vi "Arm Controller.vi"(8 "error in":errorcluster) -> ()   [LabVIEW 2019]
doc: "This VI executes continuously carrying out the current operation and responding to updates or new operations. It will often contain the timing or control code that is difficult to place directly in TeleOp. This VI generally opens all sensors and motors and isolates the rest of the robot code from knowing how the operations are carried out."
uses:
  <vilib>/Rock Robotics/WPI/Framework/Completion Status.ctl
  Arm Setpoints.ctl
  Arm Operations.ctl
  <vilib>/Rock Robotics/SystemInterfaces/DIO/FPGA_DIOChannel.ctl
  <vilib>/Rock Robotics/WPI/Encoder/WPI_EncoderType.ctl
  <vilib>/Rock Robotics/WPI/ThirdParty/Phoenix-LabVIEW/Motor Controller/Controls/CTRE_Phoenix_MotorControl_ControlMode.ctl
  <vilib>/Rock Robotics/WPI/Counter/WPI_CounterDigitalInputToDigitalSource.vi
  <vilib>/Rock Robotics/Network Tables/NT Write Boolean.vi
panel:
  in  "Interactive Values":T1
  out "Current\nCmd":string
  in  "Buttons":cluster{"Execute Cmd":bool, "Abort Cmd":bool}
  out "Command Timing":cluster{"Start Time (ms)":u32, "Iterations":i32}
  out "Status":T3
  # "Tip: It may be helpful to observe inputs and sensor values.\nYou may also want to display tuning or debugging controls."
  # "Interactive Command: You may fill in the settings for a command\nand schedule it with the Execute button. You can observe and abort\nany command while fine tuning the code for the controller."
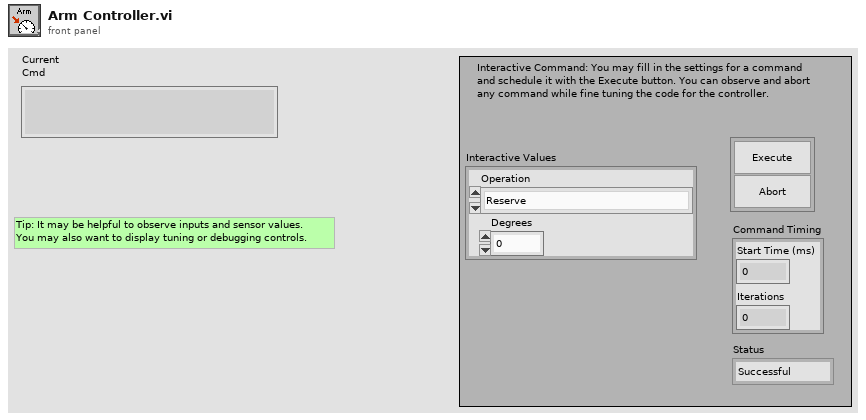
[diagram p1: front panel]
types:
  T1 = typedef "Arm Setpoints.ctl" = cluster{"Operation":T2, "Degrees":dbl}
  T2 = typedef "Arm Operations.ctl" = enum16{"Reserve", "Read Current", "bore_test", "Up", "Down", "Stop", "Up Reset", "Down Reset", "Immediate", ""}
  T3 = typedef "Completion Status.ctl" = enum16{"Successful", "Aborted", "Incomplete"}
  T4 = typedef "WPI_EncoderType.ctl" = enum16{"1x", "2x", "4x"}
  T5 = typedef "FPGA_DIOChannel.ctl" = enum8{"DIO 0", "DIO 1", "DIO 2", "DIO 3", "DIO 4", "DIO 5", "DIO 6", "DIO 7", "DIO 8", "DIO 9", "DIO MXP 0", "DIO MXP 1", "DIO MXP 2", "DIO MXP 3", "DIO MXP 4", "DIO MXP 5", "DIO MXP 6", "DIO MXP 7", "DIO MXP 8", "DIO MXP 9", "DIO MXP 10", "DIO MXP 11", "DIO MXP 12", "DIO MXP 13", "DIO MXP 14", "DIO MXP 15", "SPI Port CS1", "SPI Port CS2", "SPI Port CS3", "SPI Port MISO", "SPI Port MOSI", "Invalid"}
  T6 = typedef "WPI_MotorControlDeviceRef.ctl" = cluster{"DeviceStatus":errorcluster, "Type":T7, "PWM":cluster{"PWM Channel":T8, "DeadBand":T9}, "CAN":cluster{"Device Number":u8, "SetOutput VI Ref":variant, "GetOutput VI Ref":variant, "Enable VI Ref":variant, "Disable VI Ref":variant, "Data":variant}, "Invert":bool, "DIO PWM":cluster{"PWM \"Enable\" Channel":T8, "DIOChannel":T5, "PWM Rate":dbl}}
  T7 = typedef "WPI_MotorControlType.ctl" = enum16{"PWM", "CAN", "DIO PWM"}
  T8 = typedef "FPGA_DIOPWMChannel.ctl" = enum8{"PWM 0", "PWM 1", "PWM 2", "PWM 3", "PWM 4", "PWM 5", "PWM 6", "PWM 7", "PWM 8", "PWM 9", "PWM MXP 0", "PWM MXP 1", "PWM MXP 2", "PWM MXP 3", "PWM MXP 4", "PWM MXP 5", "PWM MXP 6", "PWM MXP 7", "PWM MXP 8", "PWM MXP 9", "Invalid"}
  T9 = typedef "WPI_PWMDeadband.ctl" = cluster{"Name":string, "maxPositivePwm":i32, "minPositivePwm":i32, "centerPwm":i32, "maxNegativePwm":i32, "minNegativePwm":i32, "angularRange":u16}
  T10 = typedef "WPI_DigitalInputDevRef.ctl" = cluster{"DevStatus":errorcluster, "DIO Channel":T5}
  T11 = typedef "FPGA_CounterEncoderSourceConvertionLVSourceType.ctl" = cluster{"DevStatus":errorcluster, "AnalogTriggerMode?":bool, "DigitalMode":cluster{"DIO Channel":T12}, "AnalogTriggerMode":cluster{"AnalogTriggerIndex":T13, "OutputType":T14}}
  T12 = typedef "FPGA_DIODigitalSourceChannel.ctl" = enum8{"DIO 0", "DIO 1", "DIO 2", "DIO 3", "DIO 4", "DIO 5", "DIO 6", "DIO 7", "DIO 8", "DIO 9", "DIO MXP 0", "DIO MXP 1", "DIO MXP 2", "DIO MXP 3", "DIO MXP 4", "DIO MXP 5", "DIO MXP 6", "DIO MXP 7", "DIO MXP 8", "DIO MXP 9", "DIO MXP 10", "DIO MXP 11", "DIO MXP 12", "DIO MXP 13", "DIO MXP 14", "DIO MXP 15", "SPI Port CS1", "SPI Port CS2", "SPI Port CS3", "SPI Port MISO", "SPI Port MOSI", "Disabled"}
  T13 = typedef "FPGA_AnalogTriggerIndex.ctl" = enum8{"Trig 0", "Trig 1", "Trig 2", "Trig 3", "Trig 4", "Trig 5", "Trig 6", "Trig 7", "Invalid"}
  T14 = typedef "FPGA_AnalogTriggerOutType.ctl" = enum16{"InWindow", "TriggerState", "Rising", "Falling"}
  T15 = typedef "WPI_EncoderDevRef.ctl" = cluster{"DevStatus":errorcluster, "EncoderIndex":T16, "CounterIndex":T17, "DistancePerCount":dbl, "Decoding Type":T4}
  T16 = typedef "FPGA_EncoderIdx.ctl" = enum8{"Enc 0", "Enc 1", "Enc 2", "Enc 3", "Enc 4", "Enc 5", "Enc 6", "Enc 7", "Invalid"}
  T17 = typedef "FPGA_CounterCtrSystemIndex.ctl" = enum8{"Ctr 0", "Ctr 1", "Ctr 2", "Ctr 3", "Ctr 4", "Ctr 5", "Ctr 6", "Ctr 7", "Invalid"}
  T18 = typedef "Command Status Info.ctl" = cluster{"Name":string, "Status":T3, "notifier out":T19}
  T19 = typedef "Completion Notifier.ctl" = refnum<notifier>
  T20 = cluster{"Current Command":T1, "Command Timing":cluster{"Start Time (ms)":u32, "Iterations":i32}, "Command Arguments":cluster{"Command Info":T18, "Description":string, "Default Command":T1, "queue out":refnum<queue>, "Subsystem Name":string}}
  T21 = typedef "CTRE_Phoenix_MotorControl_ControlMode.ctl" = u16
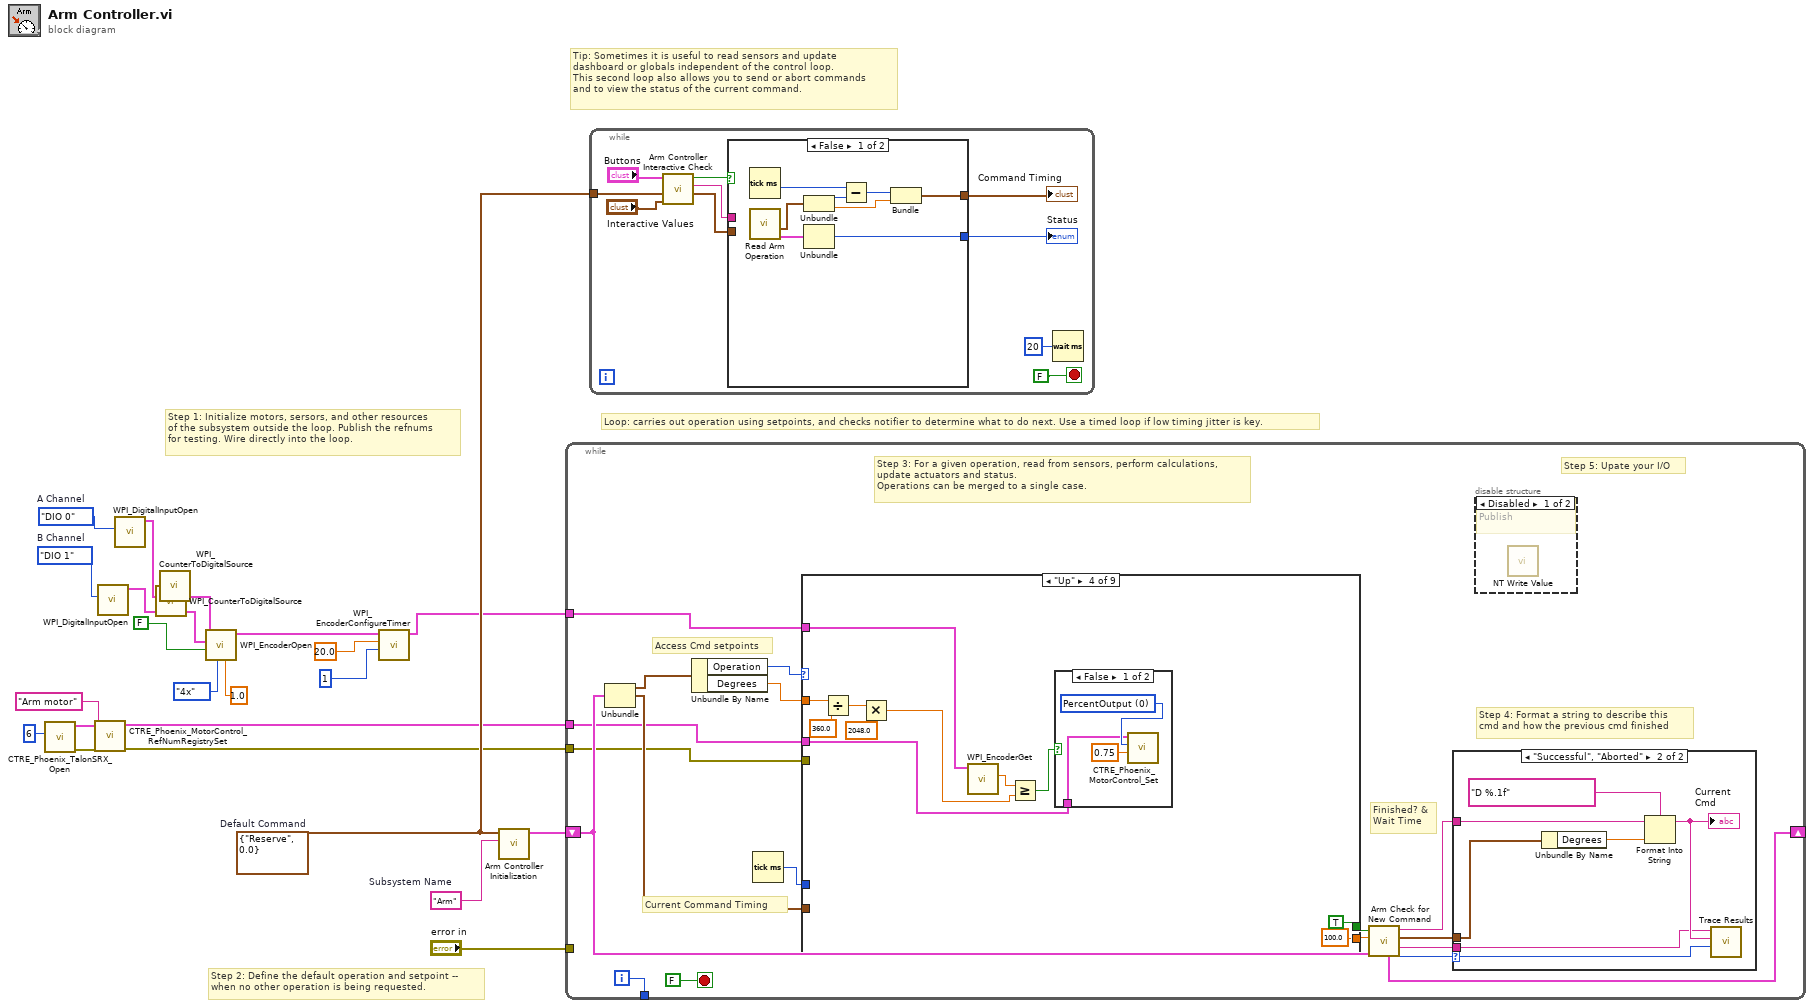
[diagram p0: block diagram]
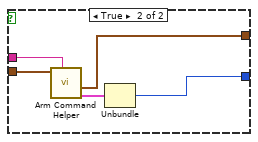
[diagram p2: hidden frame]
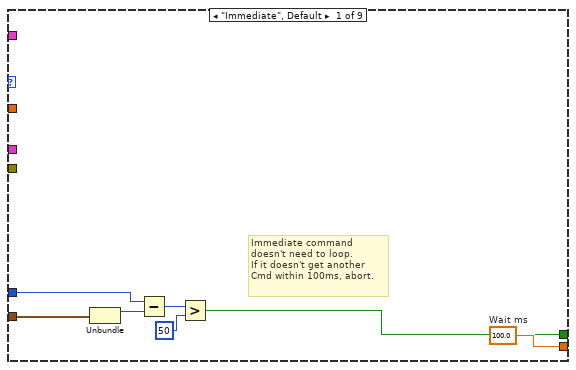
[diagram p5: hidden frame]
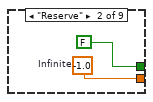
[diagram p6: hidden frame]
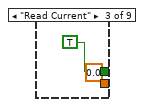
[diagram p7: hidden frame]
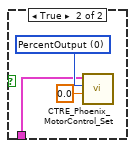
[diagram p8: hidden frame]
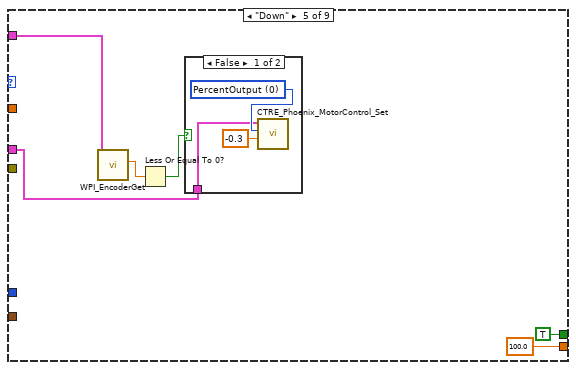
[diagram p9: hidden frame]
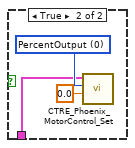
[diagram p10: hidden frame]
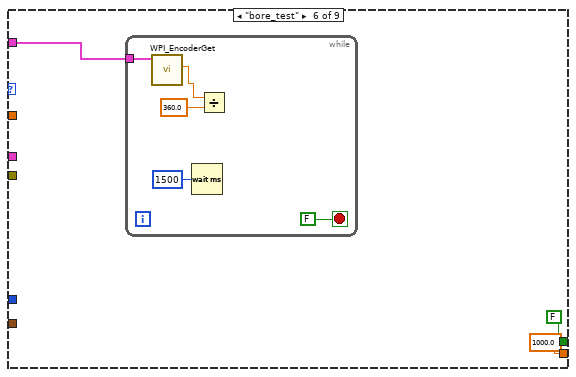
[diagram p11: hidden frame]
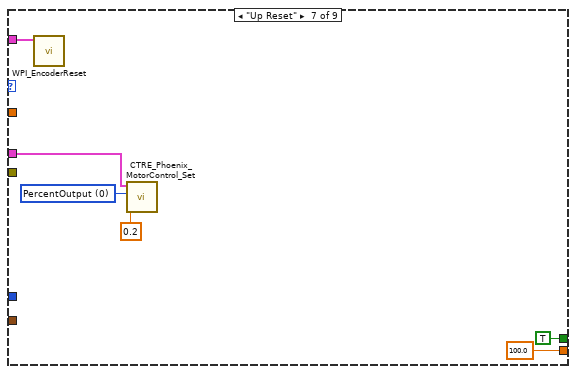
[diagram p12: hidden frame]
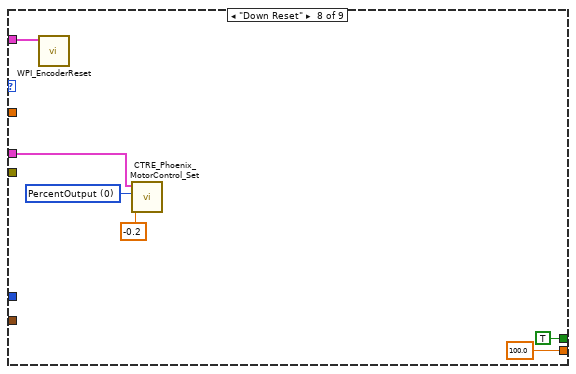
[diagram p13: hidden frame]
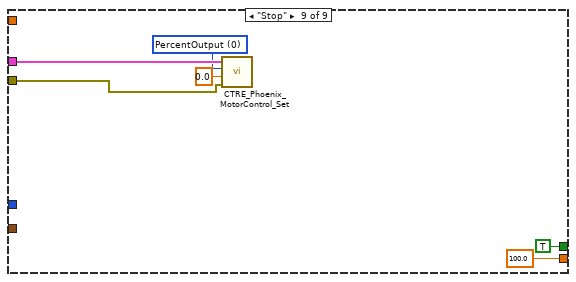
[diagram p14: hidden frame]
diagram:
  w19 = FPGA_DIOChannel."DIO 1"  # B Channel
  w18 = FPGA_DIOChannel."DIO 0"  # A Channel
  w20 = T1 {"Operation"=enum."Reserve", "Degrees"=0.0}  # Default Command
  w21 = "Arm"  # Subsystem Name
  # "Tip: Sometimes it is useful to read sensors and update\ndashboard or globals independent of the control loop.\nThis second loop also allows you to send or abort commands\nand to view the status of the current command."
  # "Step 2: Define the default operation and setpoint --\nwhen no other operation is being requested."
  # "Step 1: Initialize motors, sersors, and other resources\nof the subsystem outside the loop. Publish the refnums\nfor testing. Wire directly into the loop."
  # "Loop: carries out operation using setpoints, and checks notifier to determine what to do next. Use a timed loop if low timing jitter is key."
  n1 = call <vilib>:"CTRE_Phoenix_TalonSRX_Open.vi"("Device Number"=u8 6) -> ("error out"=w6:errorcluster, "CAN Talon SRX Ref"=w5:T6)  [unwired: 9 in]
  n2 = call <vilib>:"CTRE_Phoenix_MotorControl_RefNumRegistrySet.vi"("error in (no error)"=w6, "refnum name"="Arm motor", "PhoenixMotorControlDevRef"=w5) -> ("error out"=w2:errorcluster, "PhoenixMotorControlDevRef"=w3:T6)  [unwired: 7 in]
  n3 = call <vilib>:"WPI_DigitalInputOpen.vi"("DIO Channel"=w19) -> ("DigitalInputDevRef"=w16:T10)  [unwired: 1 in, 9 out]
  n4 = call <vilib>:"WPI_DigitalInputOpen.vi"("DIO Channel"=w18) -> ("DigitalInputDevRef"=w15:T10)  [unwired: 1 in, 9 out]
  n5 = call-poly <vilib>:"WPI_CounterToDigitalSource.vi"("DigitalInputDevRef"=w16) -> ("Digital Source"=w17:T11)  [unwired: 6 out]
  n6 = call-poly <vilib>:"WPI_CounterToDigitalSource.vi"("DigitalInputDevRef"=w15) -> ("Digital Source"=w14:T11)  [unwired: 6 out]
  n7 = call <vilib>:"WPI_EncoderOpen.vi"("DistancePerCount"=1.0, "Decoding Type"=WPI_EncoderType."4x", "Invert Direction (False)"=FALSE, "BSource"=w17, "ASource"=w14) -> ("EncoderDevRef"=w13:T15)  [unwired: 3 in, 3 out]
  n8 = call <vilib>:"WPI_EncoderConfigureTimer.vi"("Number Samples to Average"=u8 1, "Minimum Rate"=20.0, "EncoderDevRef"=w13) -> ("EncoderDevRef"=w12:T15)  [unwired: 7 in, 1 out]
  n9 = call "Arm Controller Initialization.vi"("Subsystem Name"=w21, "Default Command"=w20) -> ("Current Command"=w22:T20)  [unwired: 9 in]
  n10 = while {
    shift-right: [w36] -> _
    shift-left: w22 -> [w29]
    tunnel: [w40] -> _
    tunnel: "error in" -> [_]
    tunnel: w12 -> [w27]
    tunnel: w3 -> [w25]
    tunnel: w2 -> [w24]
    i -> [w40]
    stop <- FALSE stop-if-true
    # "Step 5: Upate your I/O"
    # "Step 4: Format a string to describe this\ncmd and how the previous cmd finished"
    # "Current Command Timing"
    # "Access Cmd setpoints"
    # "Finished? &\nWait Time"
    # "Step 3: For a given operation, read from sensors, perform calculations,\nupdate actuators and status.\nOperations can be merged to a single case."
    n11 = Unbundle(w29) -> ("Current Command"=w39:T1, "Command Timing"=w37:cluster{"Start Time (ms)":u32, "Iterations":i32})  [unwired: 1 out]
    n12 = Unbundle By Name(w39) -> ("Operation"=w26:T2, "Degrees"=w28:dbl)
    n13 = Tick Count (ms)() -> (millisecond timer value=w38:u32)
    n14 = case shown="\"Up\"" w26 {
      tunnel: [w55 w57 0.0 ("Infinite") 100.0 ("Infinite") 100.0 ("Infinite") 1000.0 ("Infinite") 100.0 ("Infinite") 100.0 ("Infinite") 100.0 ("Infinite")] -> w34
      tunnel: [w49 FALSE ("ignore previous (F)") TRUE TRUE ("ignore previous (F)") TRUE ("ignore previous (F)") FALSE ("ignore previous (F)") TRUE ("ignore previous (F)") TRUE ("ignore previous (F)") TRUE ("ignore previous (F)")] -> w35
      tunnel: w37 -> [w51 _ _ _ _ _ _ _ _]
      tunnel: w38 -> [w50 _ _ _ _ _ _ _ _]
      tunnel: w28 -> [_ _ _ w65 _ _ _ _ _]
      tunnel: w27 -> [_ _ _ w67 w80 w91 w99 w105 _]
      tunnel: w25 -> [_ _ _ w66 w79 _ w101 w106 w114]
      tunnel: w24 -> [_ _ _ _ _ _ _ _ w111]
      frame "Immediate", Default {
        w55 = 100.0  # Wait ms
        # "Immediate command\ndoesn't need to loop.\nIf it doesn't get another\nCmd within 100ms, abort."
        n15 = Unbundle(w51) -> ("Start Time (ms)"=w54:u32)  [unwired: 1 out]
        n16 = Subtract(x=w50, y=w54) -> (x-y=w53:u32)
        n17 = Greater?(x=w53, y=u8 50 ("Left Motor")) -> (0:w49:bool)
      }
      frame "Reserve" {
        w57 = -1.0  # Infinite
      }
      frame "Read Current" {
      }
      frame "Up" {
        n18 = Divide(x=w65, y=360.0) -> (x/y=w63:dbl)
        n19 = Multiply(x=w63, y=2048.0) -> (x*y=w61:dbl)
        n20 = call <vilib>:"WPI_EncoderGet.vi"("EncoderDevRef"=w67) -> ("Distance"=w69:dbl)  [unwired: 5 in, 5 out]
        n21 = Greater Or Equal?(x=w69, y=w61) -> (x >= y?=w68:bool)
        n22 = case shown="False" w68 {
          tunnel: w66 -> [w71 w74]
          frame False {
            w72 = T21 0 items=["PercentOutput"=0, "Position"=1, "Velocity"=2, "Current"=3, "Follower"=5, "MotionProfile"=6, "MotionMagic"=7, "MotionProfileArc"=10, "Disabled"=15] ("Control Mode")
            n23 = call <vilib>:"CTRE_Phoenix_MotorControl_Set.vi"("Output"=0.75, "Control Mode"=w72, "PhoenixMotorControlDevRef"=w71) -> ()  [unwired: 7 in, 2 out]
          }
          frame True {
            w76 = T21 0 items=["PercentOutput"=0, "Position"=1, "Velocity"=2, "Current"=3, "Follower"=5, "MotionProfile"=6, "MotionMagic"=7, "MotionProfileArc"=10, "Disabled"=15] ("Control Mode")
            n24 = call <vilib>:"CTRE_Phoenix_MotorControl_Set.vi"("Output"=0.0, "Control Mode"=w76, "PhoenixMotorControlDevRef"=w74) -> ()  [unwired: 7 in, 2 out]
          }
        }
      }
      frame "Down" {
        n25 = call <vilib>:"WPI_EncoderGet.vi"("EncoderDevRef"=w80) -> ("Distance"=w77:dbl)  [unwired: 5 in, 5 out]
        n26 = Less Or Equal To 0?(x=w77) -> (x <= 0?=w81:bool)
        n27 = case shown="False" w81 {
          tunnel: w79 -> [w83 w86]
          frame False {
            w84 = T21 0 items=["PercentOutput"=0, "Position"=1, "Velocity"=2, "Current"=3, "Follower"=5, "MotionProfile"=6, "MotionMagic"=7, "MotionProfileArc"=10, "Disabled"=15] ("Control Mode")
            n28 = call <vilib>:"CTRE_Phoenix_MotorControl_Set.vi"("Output"=-0.3, "Control Mode"=w84, "PhoenixMotorControlDevRef"=w83) -> ()  [unwired: 7 in, 2 out]
          }
          frame True {
            w88 = T21 0 items=["PercentOutput"=0, "Position"=1, "Velocity"=2, "Current"=3, "Follower"=5, "MotionProfile"=6, "MotionMagic"=7, "MotionProfileArc"=10, "Disabled"=15] ("Control Mode")
            n29 = call <vilib>:"CTRE_Phoenix_MotorControl_Set.vi"("Output"=0.0, "Control Mode"=w88, "PhoenixMotorControlDevRef"=w86) -> ()  [unwired: 7 in, 2 out]
          }
        }
      }
      frame "bore_test" {
        n30 = while {
          tunnel: w91 -> [w96]
          stop <- FALSE stop-if-true
          n31 = call <vilib>:"WPI_EncoderGet.vi"("EncoderDevRef"=w96) -> ("Distance"=w95:dbl)  [unwired: 5 in, 5 out]
          n32 = Wait (ms)(milliseconds to wait=u32 1500) -> ()  [unwired: 1 out]
          n33 = Divide(x=w95, y=360.0) -> ()  [unwired: 1 out]
        }
      }
      frame "Up Reset" {
        w100 = T21 0 items=["PercentOutput"=0, "Position"=1, "Velocity"=2, "Current"=3, "Follower"=5, "MotionProfile"=6, "MotionMagic"=7, "MotionProfileArc"=10, "Disabled"=15] ("Control Mode")
        n34 = call <vilib>:"WPI_EncoderReset.vi"("EncoderDevRef"=w99) -> ()  [unwired: 9 in, 2 out]
        n35 = call <vilib>:"CTRE_Phoenix_MotorControl_Set.vi"("Output"=0.2, "Control Mode"=w100, "PhoenixMotorControlDevRef"=w101) -> ()  [unwired: 7 in, 2 out]
      }
      frame "Down Reset" {
        w107 = T21 0 items=["PercentOutput"=0, "Position"=1, "Velocity"=2, "Current"=3, "Follower"=5, "MotionProfile"=6, "MotionMagic"=7, "MotionProfileArc"=10, "Disabled"=15] ("Control Mode")
        n36 = call <vilib>:"WPI_EncoderReset.vi"("EncoderDevRef"=w105) -> ()  [unwired: 9 in, 2 out]
        n37 = call <vilib>:"CTRE_Phoenix_MotorControl_Set.vi"("Output"=-0.2, "Control Mode"=w107, "PhoenixMotorControlDevRef"=w106) -> ()  [unwired: 7 in, 2 out]
      }
      frame "Stop" {
        w113 = T21 0 items=["PercentOutput"=0, "Position"=1, "Velocity"=2, "Current"=3, "Follower"=5, "MotionProfile"=6, "MotionMagic"=7, "MotionProfileArc"=10, "Disabled"=15] ("Control Mode")
        n38 = call <vilib>:"CTRE_Phoenix_MotorControl_Set.vi"("error in (no error)"=w111, "Output"=0.0, "Control Mode"=w113, "PhoenixMotorControlDevRef"=w114) -> ()  [unwired: 6 in, 2 out]
      }
    }
    n39 = call "Arm Check for New Command.vi"("Current Command"=w29, "Wait time (ms)"=w34, "Finished?"=w35) -> ("Completion"=w30:T3, "Subsystem Name"=w31:string, "Current Command"=w32:T1, "Initial Trace String"=w33:string, "NextCommand"=w36:T20)  [unwired: 4 in]
    n40 = case shown="\"Successful\", \"Aborted\"" w30 {
      selector: w30 -> [_ w48]
      tunnel: w33 -> [_ w45]
      tunnel: w32 -> [_ w46]
      tunnel: w31 -> [_ w43]
      frame "Incomplete", Default {
        # "Continuing current command"
      }
      frame "Successful", "Aborted" {
        # "Report and setup for next command"
        n41 = Unbundle By Name(w46) -> ("Degrees"=w42:dbl)
        n42 = Format Into String(format string="D %.1f", initial string=w45, w42) -> (resulting string=w44:string)  [unwired: 1 in, 1 out]
        "Current\nCmd" <- w44
        n43 = call <vilib>:"Trace Results.vi"("Status of previous command"=w48, "Description"=w44, "Subsystem"=w43) -> ()  [unwired: 9 in]
      }
    }
    n44 = disable-structure shown="Disabled" {
      frame Disabled {
        # "Publish"
        n45 = call-poly <vilib>:"NT Write Value.vi"() -> ()  [unwired: 11 in, 1 out]
      }
      frame Enabled {
      }
    }
  }
  n46 = while {
    tunnel: w20 -> [w121]
    stop <- FALSE stop-if-true
    n47 = call "Arm Controller Interactive Check.vi"("Interactive Command in"="Interactive Values", "Default Command"=w121, "Buttons"="Buttons") -> ("Interactive Command out"=w118:T1, "Trace String"=w119:string, "Schedule"=w120:bool)  [unwired: 6 in]
    n48 = case shown="False" w120 {
      tunnel: [w132 w137] -> w117
      tunnel: w118 -> [_ w135]
      tunnel: [w128 w133] -> w116
      tunnel: w119 -> [_ w136]
      frame False {
        n49 = Tick Count (ms)() -> (millisecond timer value=w127:u32)
        n50 = call "Read Arm Operation.vi"() -> ("Command Info"=w125:T18, "SubSystem Data"=w126:T1)  [unwired: 9 in, 1 out]
        n51 = Unbundle(w126) -> ("Operation"=w131:T2, "Degrees"=w129:dbl)
        n52 = Unbundle(w125) -> ("Status"=w132:T3)  [unwired: 2 out]
        n53 = Subtract(x=w127, y=w131) -> (x-y=w130:u32)
        n54 = Bundle(w130, "Degrees"=w129) -> (w128:cluster{u32, "Degrees":dbl})  [unwired: 1 in]
      }
      frame True {
        n55 = call "Arm Command Helper.vi"("Description"=w136, "SubSystem Data"=w135) -> ("Command Info Out"=w134:T18, "Command Timing"=w133:cluster{"Start Time (ms)":u32, "Iterations":i32})  [unwired: 7 in, 1 out]
        n56 = Unbundle(w134) -> ("Status"=w137:T3)  [unwired: 2 out]
      }
    }
    "Status" <- w117
    "Command Timing" <- w116
    n57 = Wait (ms)(milliseconds to wait=u32 20) -> ()  [unwired: 1 out]
  }
